vi "robot - Inner Rectangle.vi"(10 "size/2":i16=10, 11 "Rectangle In":T1) -> (3 "Rectangle Out":T1)   [LabVIEW 2023]
doc: "Given a rectangle this VI returns a square rectangle whose center is the same as the given rectangle and whose sides are twice as long as the value of the size/2 parameter. If the new rectangle is larger than the original rectangle, the original rectangle is returned in 'Rectangle Out'."
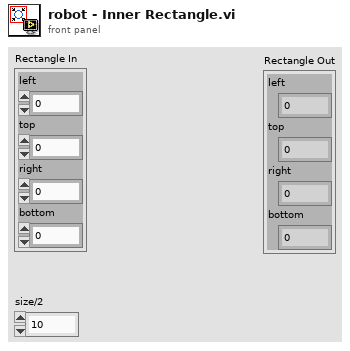
[diagram p1: front panel]
types:
  T1 = cluster{"left":i16, "top":i16, "right":i16, "bottom":i16}
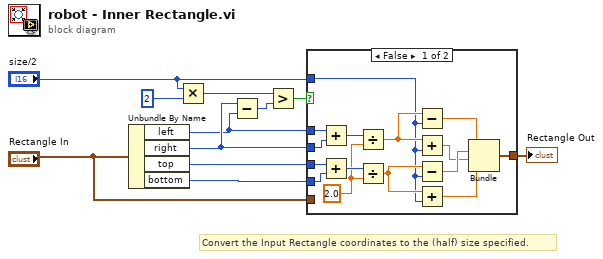
[diagram p0: block diagram]
diagram:
  # "Convert the Input Rectangle coordinates to the (half) size specified."
  n1 = Unbundle By Name("Rectangle In") -> ("left"=w7:i16, "right"=w8:i16, "top"=w9:i16, "bottom"=w11:i16)
  n2 = Multiply(x="size/2", y=i16 2) -> (x*y=w4:i16)
  n3 = Subtract(x=w8, y=w7) -> (x-y=w3:i16)
  n4 = Greater?(x=w4, y=w3) -> (0:w2:bool)
  n5 = case shown="False" w2 {
    tunnel: [w17 w27] -> w10
    tunnel: w7 -> [w26 _]
    tunnel: w8 -> [w16 _]
    tunnel: w9 -> [w15 _]
    tunnel: w11 -> [w14 _]
    tunnel: "Rectangle In" -> [_ w27]
    tunnel: "size/2" -> [w13 _]
    frame False {
      w12 = 2.0
      n6 = Add(x=w26, y=w16) -> (x+y=w19:i16)
      n7 = Add(x=w15, y=w14) -> (x+y=w18:i16)
      n8 = Divide(x=w19, y=w12) -> (x/y=w20:dbl)
      n9 = Divide(x=w18, y=w12) -> (x/y=w23:dbl)
      n10 = Subtract(x=w20, y=w13) -> (x-y=w21:dbl)
      n11 = Add(x=w20, y=w13) -> (x+y=w22:dbl)
      n12 = Subtract(x=w23, y=w13) -> (x-y=w24:dbl)
      n13 = Add(x=w23, y=w13) -> (x+y=w25:dbl)
      n14 = Bundle(w21, w24, w22, w25) -> (w17:cluster{dbl, dbl, dbl, dbl})  [unwired: 1 in]
    }
    frame True {
    }
  }
  "Rectangle Out" <- w10
